vi "mikrofon.vi"() -> ()   [LabVIEW 2017]
uses:
  C:/Users/lenovo/Source/Repos/NutkiForm/NutkiForm/bin/Debug/NutkiForm.dll
  Source/Repos/NutkiForm/NutkiForm/bin/Debug/NutkiForm.dll
  <vilib>/addons/database/Connection.llb/DB Tools Open Connec (Path).vi
  <vilib>/measure/mamon.llb/Waveform Peak Detection for N Chan.vi
  <vilib>/measure/matone.llb/Extract Single Tone Information N Chan.vi
  <vilib>/addons/database/_DB Variant To Data/Database Variant To Data.xnode
  <vilib>/measure/NI_MAPro.lvlib
  <vilib>/addons/database/NI_Database_API.lvlib
panel:
  out "# found":i32[](array[numeric])
  out "Waveform Graph 2":cluster{"Amplitudes":dbl[]}[](graph)
  out "element":string
  in  "connection information":path
  out "detected frequencies":dbl[](array[numeric]) format="%.2p"
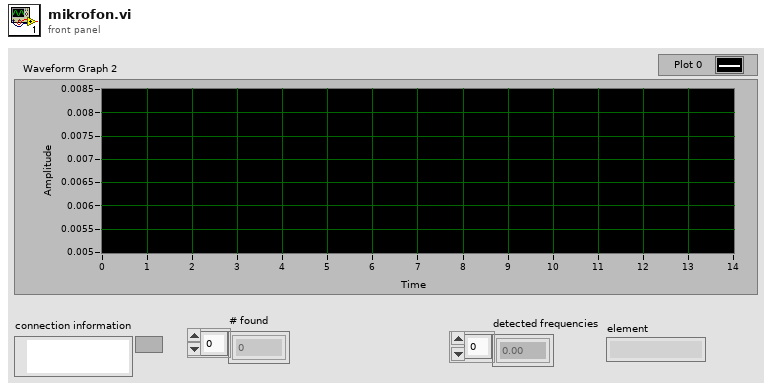
[diagram p1: front panel]
types:
  T1 = typedef "NI_Database_API.lvlib/Conn ObjectReference.ctl" = refnum<k1>
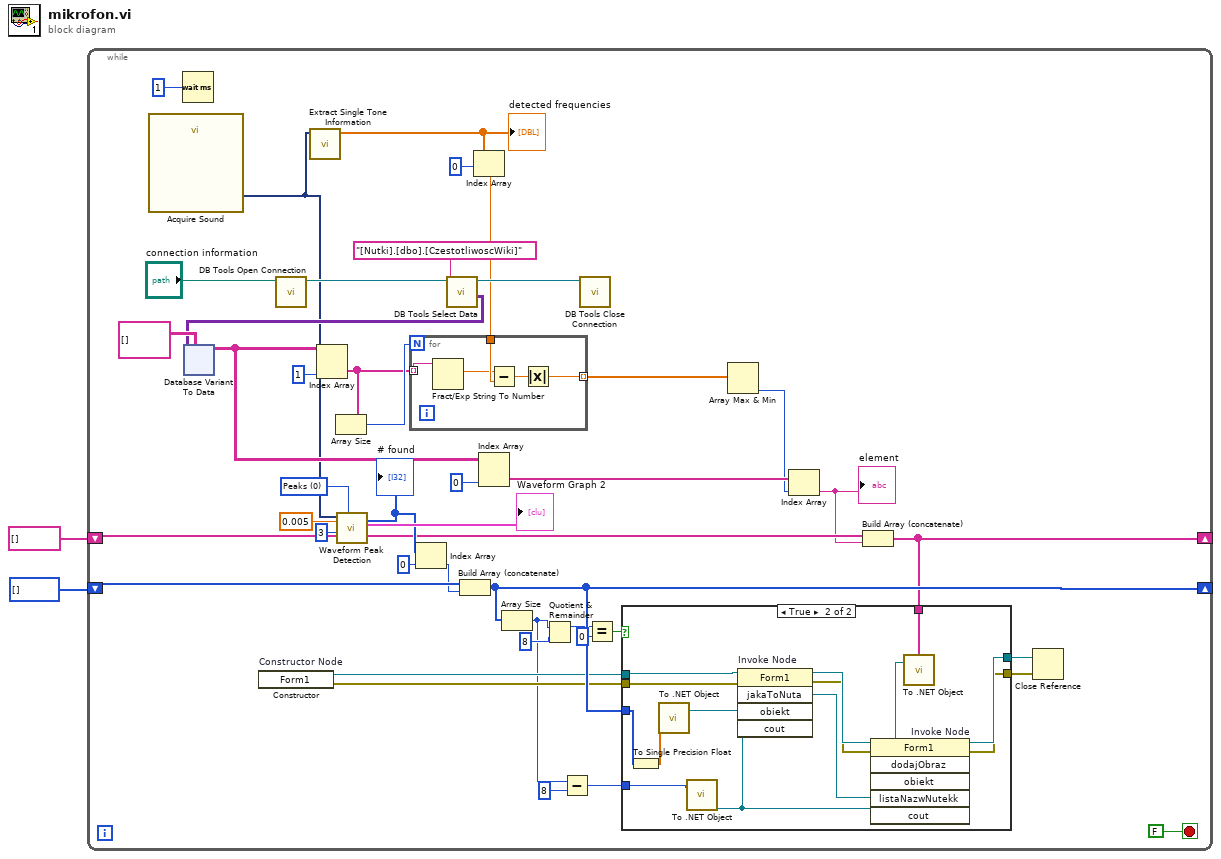
[diagram p0: block diagram]
diagram:
  n1 = while {
    shift-right: [w13] -> _
    shift-left: i32[] [] -> [w21]
    shift-right: [w10] -> _
    shift-left: string[] [] -> [w18]
    stop <- FALSE stop-if-true
    w24 = u16 0 items=["Peaks", "Valleys"] ("peaks/valleys")
    n2 = call "Acquire Sound"() -> ("Data"=w26:dynamicdata)  [unwired: 18 in, 1 out]
    n3 = Wait (ms)(milliseconds to wait=u32 1) -> ()  [unwired: 1 out]
    n4 = constructor on="Constructor Node" class="Form1"() -> (reference out=w12:refnum<k24>, error out=w11:errorcluster)  [unwired: 3 in, 1 out]
    n5 = call-poly <vilib>:"DB Tools Open Connection.vi"("connection information"="connection information") -> ("connection reference"=w42:T1)  [unwired: 7 in, 1 out]
    n6 = call-poly <vilib>:"Extract Single Tone Information.vi"("time signals in"=w26) -> ("detected frequencies"=w30:dbl[])  [unwired: 5 in, 5 out]
    "detected frequencies" <- w30
    n7 = call-poly <vilib>:"Waveform Peak Detection.vi"("peaks/valleys"=w24, "width"=3, "threshold"=0.005, "Signals In"=w26) -> ("Amplitudes"=→"Waveform Graph 2":cluster{"Amplitudes":dbl[]}[], "# found"=w20:i32[])  [unwired: 3 in, 3 out]
    "# found" <- w20
    n8 = Index Array "Index Array"(array=w20, index=0) -> (element=w16:i32)
    n9 = call <vilib>:"DB Tools Select Data.vi"("table"="[Nutki].[dbo].[CzestotliwoscWiki]", "connection reference"=w42) -> ("data"=w37:variant[][], "connection reference out"=w41:T1)  [unwired: 4 in, 1 out]
    n10 = xnode "Database Variant To Data"("database variant"=w37, "type"=string[][] []) -> ("data"=w34:string[][])  [unwired: 1 in, 1 out]
    n11 = Index Array "Index Array"(array=w34, index (col)=1 ("disabled index (col)")) -> (element=w35:string[])  [unwired: 1 in]
    n12 = Array Size(array=w35) -> (size(s)=w39:i32)
    n13 = Build Array (concatenate) "Build Array"(w21, w16) -> (w13:i32[])
    n14 = Index Array(array=w30, index=0) -> (element=w28:dbl)
    n15 = for {
      N: w39 -> [_]
      tunnel: w35 -> [w108] mode=indexing
      tunnel: [w109] -> w31 mode=indexing
      tunnel: w28 -> [w107]
      n16 = Fract/Exp String To Number(string=w108) -> (number=w106:dbl)  [unwired: 3 in, 1 out]
      n17 = Subtract(x=w106, y=w107) -> (x-y=w110:dbl)
      n18 = Absolute Value(x=w110) -> (abs(x)=w109:dbl)
    }
    n19 = Index Array "Index Array"(array=w34, index (col)=0 ("disabled index (col)")) -> (element=w32:string[])  [unwired: 1 in]
    n20 = Array Size(array=w13) -> (size(s)=w5:i32)
    n21 = Quotient & Remainder(x=w5, y=8) -> (x-y*floor(x/y)=w7:i32)  [unwired: 1 out]
    n22 = Subtract(x=w5, y=8) -> (x-y=w3:i32)
    n23 = call <vilib>:"DB Tools Close Connection.vi"("connection reference"=w41) -> ()  [unwired: 6 in, 1 out]
    n24 = Equal?(x=w7, y=0) -> (x = y?=w8:bool)
    n25 = Array Max & Min(array=w31) -> (min index (indices)=w27:i32)  [unwired: 3 out]
    n26 = Index Array "Index Array"(array=w32, index=w27) -> (element=w17:string)
    "element" <- w17
    n27 = Build Array (concatenate) "Build Array"(w18, w17) -> (w10:string[])
    n28 = case shown="True" w8 {
      tunnel: [w47 w61] -> w15
      tunnel: [w46 w60] -> w14
      tunnel: w13 -> [_ w51]
      tunnel: w12 -> [w47 w59]
      tunnel: w11 -> [w46 w58]
      tunnel: w10 -> [_ w56]
      tunnel: w3 -> [_ w49]
      frame False {
      }
      frame True {
        n29 = To Single Precision Float(number=w51) -> (single precision float=w50:sgl[])
        n30 = call <vilib>:"To .NET Object.vi"("anything"=w50) -> (".NET object"=w53:refnum<k24>)  [unwired: 1 in, 1 out]
        n31 = call <vilib>:"To .NET Object.vi"("anything"=w49) -> (".NET object"=w48:refnum<k24>)  [unwired: 1 in, 1 out]
        n32 = invoke on="Invoke Node" class="Form1" method="jakaToNuta"(reference=w59, error in=w58, "obiekt"=w53, "cout"=w48) -> (reference out=w55:refnum<k24>, error out=w54:errorcluster, "jakaToNuta"=w57:refnum<k24>)  [unwired: 1 in, 2 out]
        n33 = call <vilib>:"To .NET Object.vi"("anything"=w56) -> (".NET object"=w52:refnum<k24>)  [unwired: 1 in, 1 out]
        n34 = invoke on="Invoke Node" class="Form1" method="dodajObraz"(reference=w55, error in=w54, "obiekt"=w52, "listaNazwNutekk"=w57, "cout"=w48) -> (reference out=w61:refnum<k24>, error out=w60:errorcluster)  [unwired: 1 in, 4 out]
      }
    }
    n35 = Close Reference(reference=w15, error in (no error)=w14) -> ()  [unwired: 1 out]
  }
